vi "Update Frame Element Before Kalman.vi"(10 "Old Array With Kalman":T1[](array[typedef]) {"robots_blue"."height" format="%+4.3f"; "robots_blue"."pixel_y" format="%+4.3f"; "robots_blue"."pixel_x" format="%+4.3f"; "robots_blue"."orientation" format="%+4.3f"; "robots_blue"."y" format="%+4.3f"; "robots_blue"."confidence" format="%4.3f"; "robots_blue"."x" format="%+4.3f"; "robots_yellow"."height" format="%+4.3f"; "robots_yellow"."pixel_y" format="%+4.3f"; "robots_yellow"."pixel_x" format="%+4.3f"; "robots_yellow"."orientation" format="%+4.3f"; "robots_yellow"."y" format="%+4.3f"; "robots_yellow"."confidence" format="%4.3f"; "robots_yellow"."x" format="%+4.3f"}, 11 "New Array":T1[](array[typedef]) {"robots_blue"."height" format="%+4.3f"; "robots_blue"."pixel_y" format="%+4.3f"; "robots_blue"."pixel_x" format="%+4.3f"; "robots_blue"."orientation" format="%+4.3f"; "robots_blue"."y" format="%+4.3f"; "robots_blue"."confidence" format="%4.3f"; "robots_blue"."x" format="%+4.3f"; "robots_yellow"."height" format="%+4.3f"; "robots_yellow"."pixel_y" format="%+4.3f"; "robots_yellow"."pixel_x" format="%+4.3f"; "robots_yellow"."orientation" format="%+4.3f"; "robots_yellow"."y" format="%+4.3f"; "robots_yellow"."confidence" format="%4.3f"; "robots_yellow"."x" format="%+4.3f"}) -> (3 "Detection Frame In out":T1[](array[typedef]) {"robots_blue"."height" format="%+4.3f"; "robots_blue"."pixel_y" format="%+4.3f"; "robots_blue"."pixel_x" format="%+4.3f"; "robots_blue"."orientation" format="%+4.3f"; "robots_blue"."y" format="%+4.3f"; "robots_blue"."confidence" format="%4.3f"; "robots_blue"."x" format="%+4.3f"; "robots_yellow"."height" format="%+4.3f"; "robots_yellow"."pixel_y" format="%+4.3f"; "robots_yellow"."pixel_x" format="%+4.3f"; "robots_yellow"."orientation" format="%+4.3f"; "robots_yellow"."y" format="%+4.3f"; "robots_yellow"."confidence" format="%4.3f"; "robots_yellow"."x" format="%+4.3f"})   [LabVIEW 2017]
uses:
  SSL Detection Frame.ctl
  SSL Detection Robot.ctl
  <vilib>/Analysis/Matrix/Datatypes/RealMatrix.ctl
  SSL Detection Ball.ctl
  <vilib>/Analysis/Matrix/NI_Matrix.lvlib
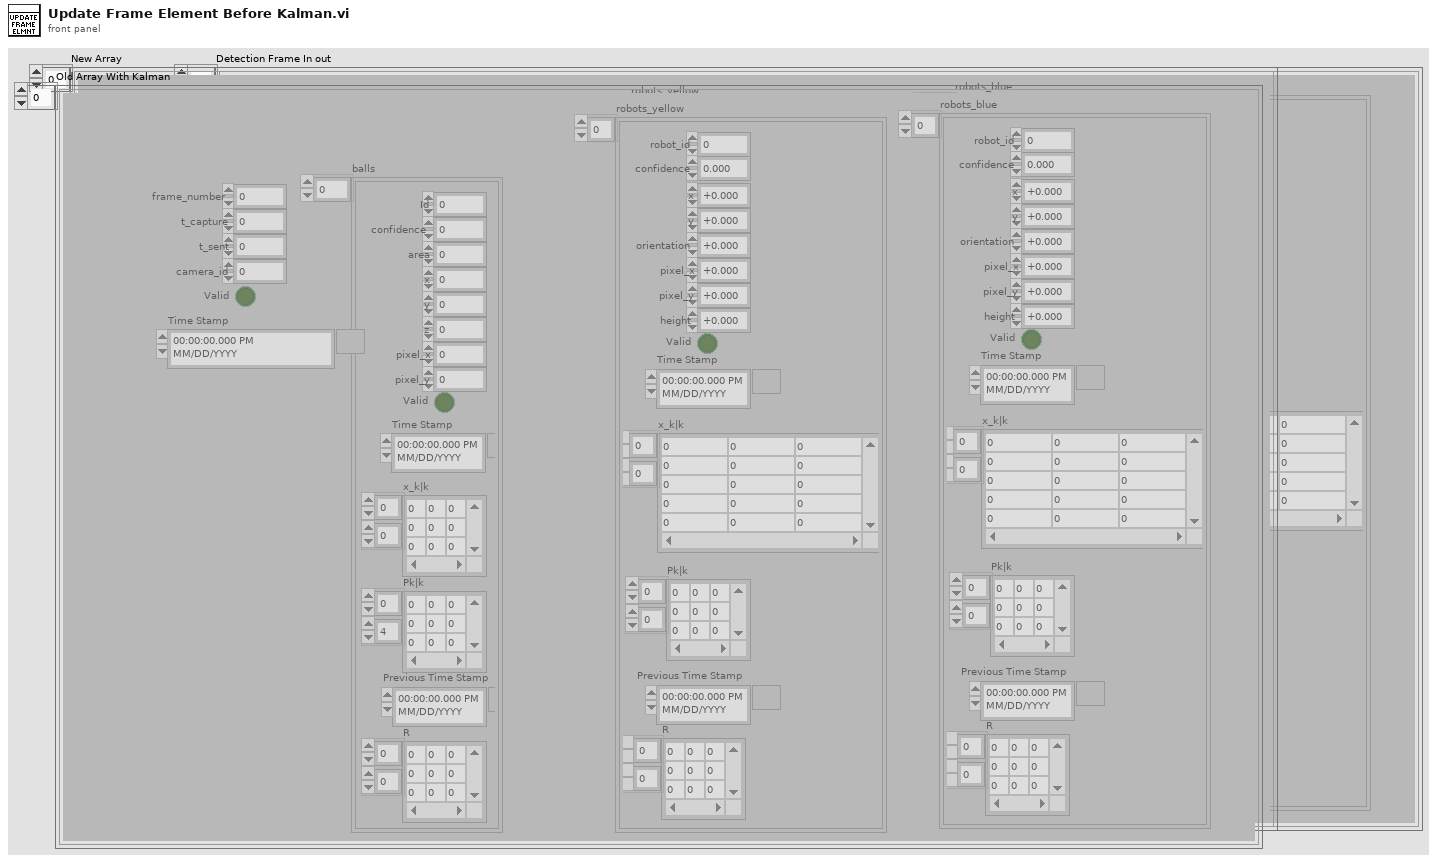
[diagram p1: front panel]
types:
  T1 = typedef "SSL Detection Frame.ctl" = cluster{"frame_number":u32, "t_capture":dbl, "t_sent":dbl, "camera_id":u32, "robots_yellow":T2[], "robots_blue":T2[], "balls":T4[], "Valid":bool, "Time Stamp":timestamp}
  T2 = typedef "SSL Detection Robot.ctl" = cluster{"x":sgl, "robot_id":u32, "confidence":sgl, "y":sgl, "orientation":sgl, "pixel_x":sgl, "pixel_y":sgl, "height":sgl, "Valid":bool, "Time Stamp":timestamp, "x_k|k":T3, "Pk|k":T3, "Previous Time Stamp":timestamp, "R":T3}
  T3 = typedef "NI_Matrix.lvlib/RealMatrix.ctl" = dbl[][]
  T4 = typedef "SSL Detection Ball.ctl" = cluster{"x":sgl, "area":u32, "confidence":sgl, "y":sgl, "z":sgl, "pixel_x":sgl, "pixel_y":sgl, "Valid":bool, "Time Stamp":timestamp, "x_k|k":T3, "Pk|k":T3, "Id":u32, "Previous Time Stamp":timestamp, "R":T3}
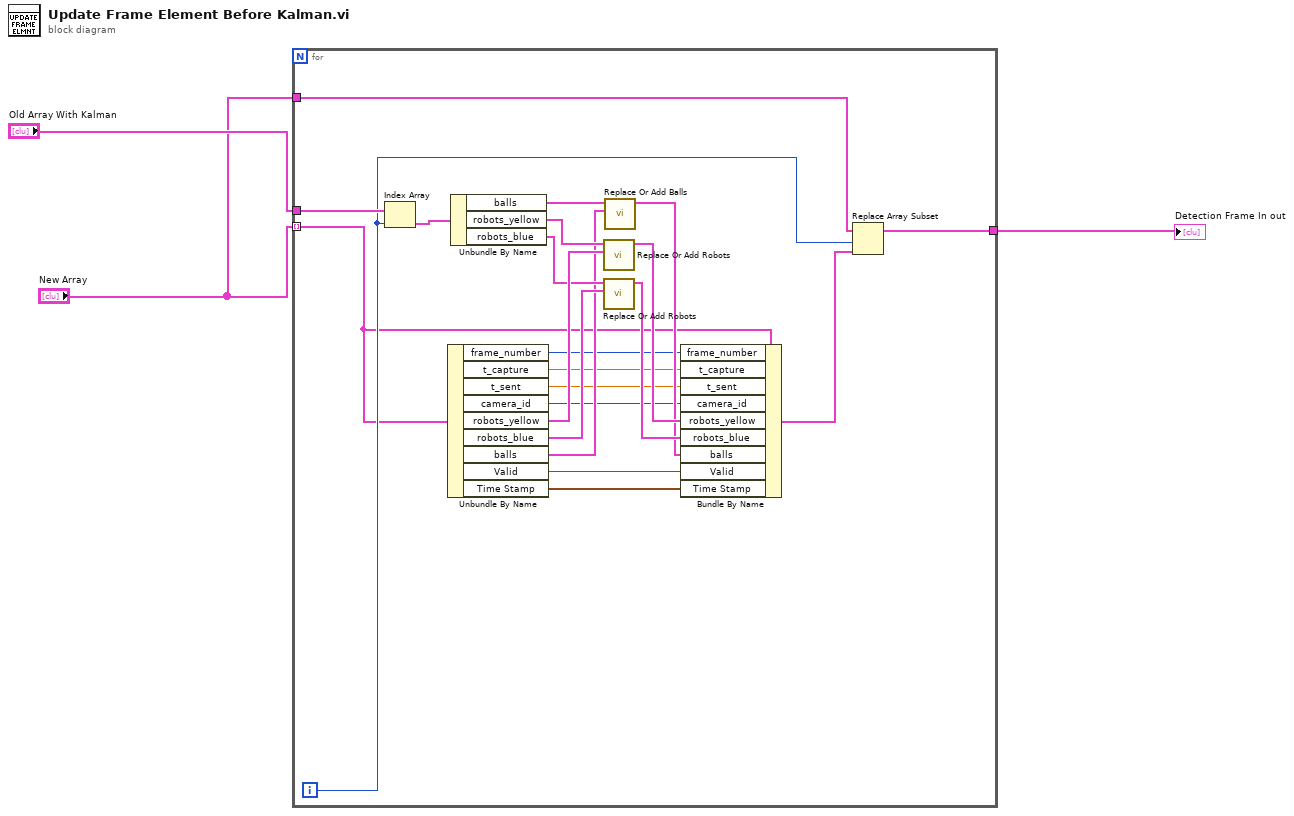
[diagram p0: block diagram]
diagram:
  n1 = for {
    tunnel: [w25] -> w3
    tunnel: "New Array" -> [w5] mode=indexing
    tunnel: "Old Array With Kalman" -> [w24]
    tunnel: "New Array" -> [w4]
    i -> [w12]
    n2 = Index Array(array=w24, index=w12) -> (element=w23:T1)
    n3 = Unbundle By Name(w5) -> ("frame_number"=w11:u32, "t_capture"=w10:dbl, "t_sent"=w9:dbl, "camera_id"=w8:u32, "robots_yellow"=w21:T2[], "robots_blue"=w18:T2[], "balls"=w14:T4[], "Valid"=w7:bool, "Time Stamp"=w6:timestamp)
    n4 = Unbundle By Name(w23) -> ("balls"=w15:T4[], "robots_yellow"=w22:T2[], "robots_blue"=w19:T2[])
    n5 = call "Replace Or Add Robots.vi"("Robots New"=w21, "Robots Old"=w22) -> ("Robots New Out"=w20:T2[])  [unwired: 9 in]
    n6 = call "Replace Or Add Robots.vi"("Robots New"=w18, "Robots Old"=w19) -> ("Robots New Out"=w17:T2[])  [unwired: 9 in]
    n7 = call "Replace Or Add Balls.vi"("balls new"=w14, "balls"=w15) -> ("Balls out"=w13:T4[])  [unwired: 9 in]
    n8 = Bundle By Name(cluster=w5, "frame_number"=w11, "t_capture"=w10, "t_sent"=w9, "camera_id"=w8, "robots_yellow"=w20, "robots_blue"=w17, "balls"=w13, "Valid"=w7, "Time Stamp"=w6) -> (w16:T1)
    n9 = Replace Array Subset(array=w4, new element=w16, index=w12) -> (w25:T1[])
  }
  "Detection Frame In out" <- w3
